vi "_Noise_YIG3.vi"(5 "Noise_YIG":T3={"Start(GHz)"=3.8, "Stop(GHz)"=12.2, "Step(GHz) "=0.2, "wait (S)"=0.1, "H/C SW"=0, "file_name"="", "P.M.aveg"=10, "save"=TRUE} {"H/C SW" items=["Liq Ni Motor", "NoiseSource Pow", "NoiseSource SP4T SW"]}, 6 "Bias_LO_equip":T1={"Node address"=19, "CAN Interface"="CAN1", "Cartridge band"=10, "Slave Node in"={"Address"=19, "Serial Number"=[16, 71, 55, 76, 1, 8, 0, -15]}, "ObjHandle out"=176554048, "POL"=1, "sb"=1, "GPIB_SM (SIS S,V)"="24", "GPIB_DMM (SIS I)"="22", "GPIB_SM (MAG I) "="25", "GPIB_SG(LO)"="19", "GPIB_PW (PAMP) "="6", "GPIB_TMP1(8ch)"="12", "GPIB_TMP2(2ch)  "="13", "WCA_avg"=10, "Rsen"=10.0, "BiasModule"=1, "LOModule "=5, "WCA_LO_FREQ_SET"={"YTO Low freq. [GHz]"=14.42, "YTO High freq. [GHz]"=17.7, "Kvco"=1, "Lock Pol."=0, "SET LO FREQ"=96.22222, "Multiplier"=6.0, "YTO (HEX)"=2014, "YTO ( FREQ)"=16.033167, "NULL PLL INTEGRATOR"=FALSE}, "Res for"=0} {"Res for" items=["none", "series res", "parallel res"]; "WCA_LO_FREQ_SET"."YTO ( FREQ)" min=25 max=150 step=0.0001 format="%.3f"; "WCA_LO_FREQ_SET"."Multiplier" min=3 max=6 step=3; "WCA_LO_FREQ_SET"."SET LO FREQ" min=25 max=150 step=0.0001 format="%.3f"; "WCA_LO_FREQ_SET"."Lock Pol." items=["Lower", "Upper"]; "WCA_LO_FREQ_SET"."Kvco" items=["7.5MHz/V", "15MHz/V"]; "WCA_LO_FREQ_SET"."YTO High freq. [GHz]" format="%.3f"; "WCA_LO_FREQ_SET"."YTO Low freq. [GHz]" format="%.3f"; "LOModule" items=["Manual Gunn+PAMP"=0, "PLL GUNN+PAMP"=5, "B10Lab LO"=1, "WCA LO"=2, ""=3, "YIG発信器"=4, "none"=99]; "BiasModule" items=["B10Lab Bias"=0, "WCA BiasModule"=1, "none"=99]; "Slave Node in"."Serial Number" format="%.0x"; "Slave Node in"."Address" format="%.0x"; "Cartridge band" max=10 step=1; "Node address" format="%.0x"}, 7 "Control":T2={"GPIB_ATT"="28", "6501Dev#"=1, "GPIB_SP"="18", "GPIB_PM"="13", "GPIB_DSA"="11", "GPIB_DMM (TPD)"="23", "GPIB_MPI"="2", "mortor設定"=[{"Axis"=0, "ID"=0, "HIspeed"=200.0, "LOspeed"=100.0, "ACCEL(ms)"=100.0, "Sratio"=50.0, "フリーラン\n"=FALSE, "文字列"="DSB HOT/COLD"}, {"Axis"=1, "ID"=0, "HIspeed"=4.0, "LOspeed"=4.0, "ACCEL(ms)"=100.0, "Sratio"=50.0, "フリーラン\n"=TRUE, "文字列"="SubMM Att"}, {"Axis"=0, "ID"=0, "HIspeed"=200.0, "LOspeed"=100.0, "ACCEL(ms)"=100.0, "Sratio"=50.0, "フリーラン\n"=TRUE, "文字列"="MPI Port1"}, {"Axis"=1, "ID"=0, "HIspeed"=200.0, "LOspeed"=100.0, "ACCEL(ms)"=100.0, "Sratio"=50.0, "フリーラン\n"=TRUE, "文字列"="MPI Port2"}], "DATAパス"=path "C:/Documents and Settings/?澤佳?/デスクトップ/data/プロトカ?トリッジ/100811_protC4-5/100904_P1_WCA_YIG", "DBパス "=path "Z:/band10/Labview_ALMA/MIX95/test", "comment"="100904_P1", "ColdCarts"="003601", "Th"=295.0, "Tc"=77.0, "Set_SIS_volt"=2.056451612903226, "Offset"=0.0, "control"=0, "FreqLO"=866.0, "Set_Mag_Cur"=800.0, "MPI offset(mm)"=22.986, "HOT/COLD"=0} {"HOT/COLD" items=["DSB", "SBR (Cart.)", "GainComp", "SBR (MIX)"]; "control" items=["CLOSE LOOP", "OPEN LOOP", "Not Control"]}) -> ()   [LabVIEW 2017]
uses:
  <vilib>/express/express arith-compare/Formula/XNode/ExpressFormulaBlockNode.xnode
panel:
  out "文字列":string
  in  "GPIB_NSPOW":string="4"
  out "XYグラフ 2":cluster{dbl[], dbl[]}(graph)={[3.8, 4.0, 4.2, 4.4, 4.6000000000000005, 4.800000000000001, 5.000000000000001, 5.200000000000001, 5.400000000000001, 5.600000000000001, 5.800000000000002, 6.000000000000002, 6.200000000000002, 6.400000000000002, 6.600000000000002, 6.8000000000000025, 7.000000000000003, 7.200000000000003, 7.400000000000003, 7.600000000000003, 7.800000000000003, 8.000000000000004, 8.200000000000003, 8.400000000000002, 8.600000000000001, 8.8, 9.0, 9.2, 9.399999999999999, 9.599999999999998, 9.799999999999997, 9.999999999999996, 10.199999999999996, 10.399999999999995, 10.599999999999994, 10.799999999999994, 10.999999999999993, 11.199999999999992, 11.399999999999991, 11.59999999999999, 11.79999999999999, 11.99999999999999, 12.199999999999989], [2162.2506307736817, 2610.001590658997, 3259.5497781050235, 2775.320412397087, 1731.9983281356488, 2481.779183137006, 2157.7510673198776, 1361.8845474426378, 682.5925239823699, 467.0395463865505, 435.3183157956642, 349.7678766673094, 257.35595108351663, 289.17415724926303, 272.2311885625452, 209.59141580739004, 206.53463871352125, 209.82364143887986, 193.6852217403505, 194.85552081739866, 186.2536165476463, 179.66627306574705, 180.29108492826452, 165.88232684665306, 170.21484313825314, 165.08707486423583, 161.69317508275617, 161.39594860807668, 157.61356167006898, 158.36459186549865, 162.3085451942526, 161.9946346155518, 165.27352115402942, 175.3117039214409, 165.6089313162741, 172.40460358258508, 178.15219547665433, 172.86473012765347, 183.70006104814289, 180.09761807812546, 191.78147420273163, 202.2277082874304, 182.5702492273905]}
  out "XYグラフ":cluster{dbl[], dbl[]}[](graph)=[{[3.8, 4.0, 4.2, 4.4, 4.6000000000000005, 4.800000000000001, 5.000000000000001, 5.200000000000001, 5.400000000000001, 5.600000000000001, 5.800000000000002, 6.000000000000002, 6.200000000000002, 6.400000000000002, 6.600000000000002, 6.8000000000000025, 7.000000000000003, 7.200000000000003, 7.400000000000003, 7.600000000000003, 7.800000000000003, 8.000000000000004, 8.200000000000003, 8.400000000000002, 8.600000000000001, 8.8, 9.0, 9.2, 9.399999999999999, 9.599999999999998, 9.799999999999997, 9.999999999999996, 10.199999999999996, 10.399999999999995, 10.599999999999994, 10.799999999999994, 10.999999999999993, 11.199999999999992, 11.399999999999991, 11.59999999999999, 11.79999999999999, 11.99999999999999, 12.199999999999989], [-12.6875455, -8.79275512, -6.28005577, -6.92868098, -8.7166628, -7.23493494, -7.37364738, -9.71131351, -11.7554011, -12.0808461, -12.5492271, -12.7463133, -13.372812, -14.3472225, -14.8493371, -15.5347475, -15.4508156, -15.5883011, -15.8732176, -15.6557263, -15.5366824, -16.038689, -16.8987194, -16.5991598, -17.7414209, -17.8823822, -17.4270802, -18.165907, -17.9285973, -17.7668847, -18.7346471, -18.8135922, -20.0978527, -20.2293386, -19.0504215, -19.9008061, -19.8130024, -19.1671194, -20.4106312, -20.1865464, -20.5863901, -22.2963949, -21.6268169]}, {[3.8, 4.0, 4.2, 4.4, 4.6000000000000005, 4.800000000000001, 5.000000000000001, 5.200000000000001, 5.400000000000001, 5.600000000000001, 5.800000000000002, 6.000000000000002, 6.200000000000002, 6.400000000000002, 6.600000000000002, 6.8000000000000025, 7.000000000000003, 7.200000000000003, 7.400000000000003, 7.600000000000003, 7.800000000000003, 8.000000000000004, 8.200000000000003, 8.400000000000002, 8.600000000000001, 8.8, 9.0, 9.2, 9.399999999999999, 9.599999999999998, 9.799999999999997, 9.999999999999996, 10.199999999999996, 10.399999999999995, 10.599999999999994, 10.799999999999994, 10.999999999999993, 11.199999999999992, 11.399999999999991, 11.59999999999999, 11.79999999999999, 11.99999999999999, 12.199999999999989], [-13.091013, -9.13153963, -6.55492569, -7.24853488, -9.21081505, -7.5900203, -7.77789058, -10.3239765, -12.851173, -13.5443165, -14.0889502, -14.53843, -15.5529118, -16.375769, -16.9558079, -17.9915143, -17.9277637, -18.0435485, -18.4388642, -18.2130248, -18.156679, -18.7088847, -19.5640687, -19.3811012, -20.4872111, -20.6710665, -20.2449254, -20.9863361, -20.7823418, -20.6139494, -21.5471582, -21.6288217, -22.8849531, -22.9338225, -21.8346772, -22.6286913, -22.4950179, -21.8912729, -23.0498547, -22.8533944, -23.1657372, -24.802363, -24.2746404]}]
  # "ENR21.8=>44183K"
  # "HOT/COLDのNoiseSourcePow\nはケンウッド電源のON/OFFのみ\n電圧は手動で設定する。"
  # "LO freq. [GHz]"
  # "YTO LOW\n/High Freq."
  # "ZERO Intgrtr"
  # "Node Address"
  # "Serial Number"
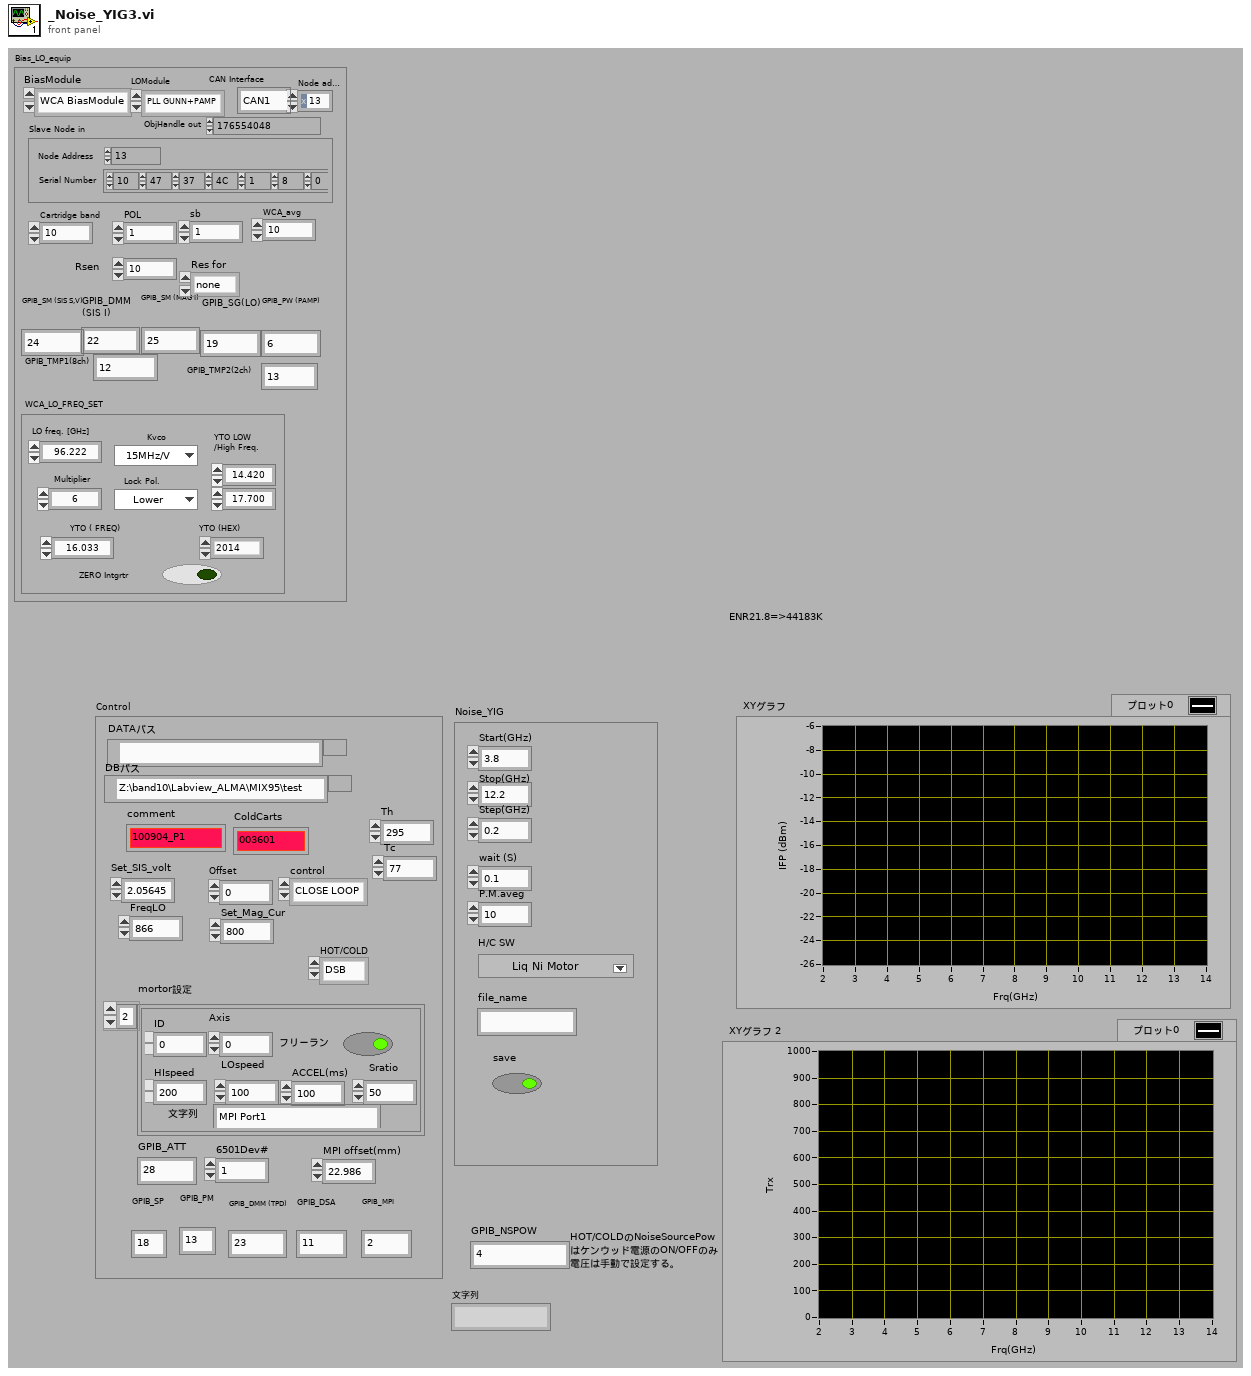
[diagram p1: front panel]
types:
  T1 = cluster{"Node address":u16, "CAN Interface":string, "Cartridge band":u32, "Slave Node in":cluster{"Address":i16, "Serial Number":i8[]}, "ObjHandle out":u32, "POL":u32, "sb":u32, "GPIB_SM (SIS S,V)":string, "GPIB_DMM (SIS I)":string, "GPIB_SM (MAG I) ":string, "GPIB_SG(LO)":string, "GPIB_PW (PAMP) ":string, "GPIB_TMP1(8ch)":string, "GPIB_TMP2(2ch)  ":string, "WCA_avg":i32, "Rsen":dbl, "BiasModule":u16, "LOModule ":u16, "WCA_LO_FREQ_SET":cluster{"YTO Low freq. [GHz]":sgl, "YTO High freq. [GHz]":sgl, "Kvco":u16, "Lock Pol.":u16, "SET LO FREQ":sgl, "Multiplier":sgl, "YTO (HEX)":u16, "YTO ( FREQ)":sgl, "NULL PLL INTEGRATOR":bool}, "Res for":u16}
  T2 = cluster{"GPIB_ATT":string, "6501Dev#":i16, "GPIB_SP":string, "GPIB_PM":string, "GPIB_DSA":string, "GPIB_DMM (TPD)":string, "GPIB_MPI":string, "mortor設定":cluster{"Axis":i16, "ID":i16, "HIspeed":dbl, "LOspeed":dbl, "ACCEL(ms)":dbl, "Sratio":dbl, "フリーラン\n":bool, "文字列":string}[], "DATAパス":path, "DBパス ":path, "comment":string, "ColdCarts":string, "Th":dbl, "Tc":dbl, "Set_SIS_volt":dbl, "Offset":dbl, "control":u16, "FreqLO":dbl, "Set_Mag_Cur":dbl, "MPI offset(mm)":dbl, "HOT/COLD":u16}
  T3 = cluster{"Start(GHz)":dbl, "Stop(GHz)":dbl, "Step(GHz) ":dbl, "wait (S)":dbl, "H/C SW":u16, "file_name":string, "P.M.aveg":i32, "save":bool}
  T4 = cluster{"Axis":i16, "ID":i16, "HIspeed":dbl, "LOspeed":dbl, "ACCEL(ms)":dbl, "Sratio":dbl, "フリーラン\n":bool, "文字列":string}[]
  T5 = cluster{"Axis":i16, "ID":i16, "HIspeed":dbl, "LOspeed":dbl, "ACCEL(ms)":dbl, "Sratio":dbl, "フリーラン\n":bool, "文字列":string}
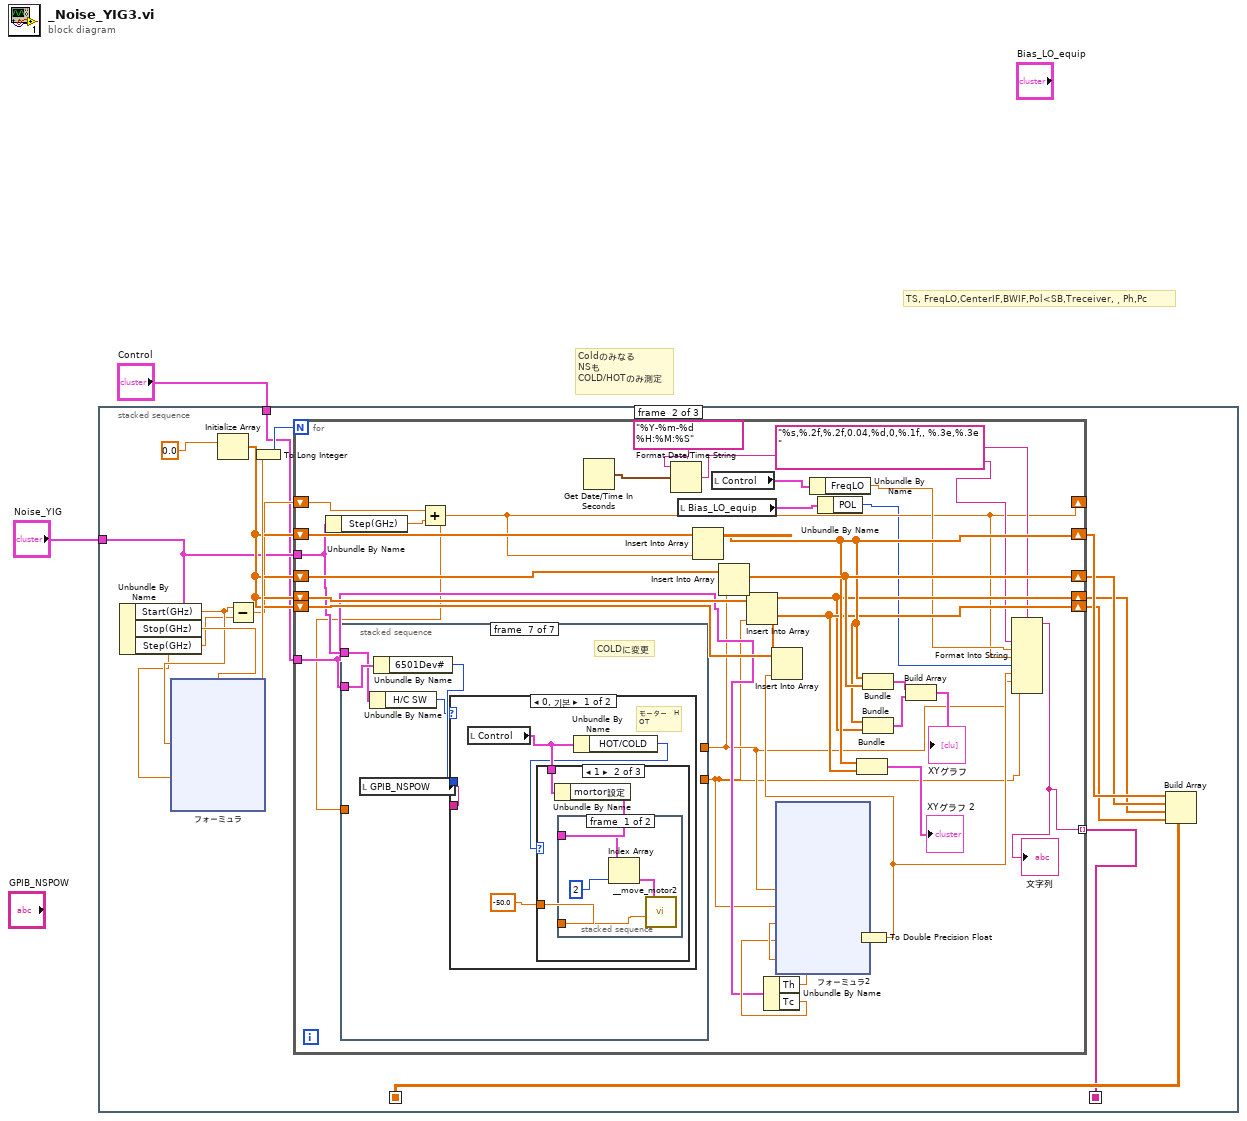
[diagram p0: block diagram]
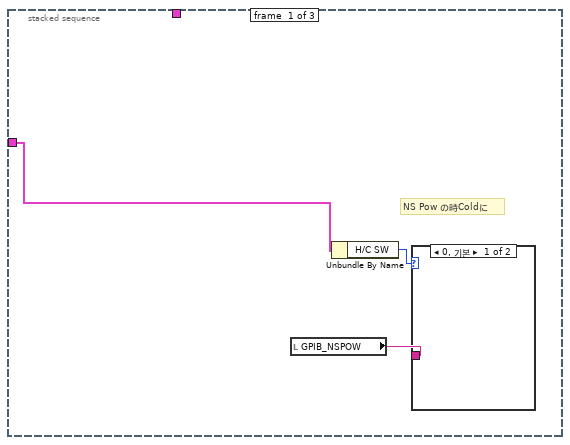
[diagram p2: hidden frame]
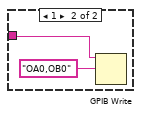
[diagram p3: hidden frame]
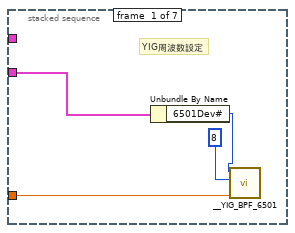
[diagram p4: hidden frame]
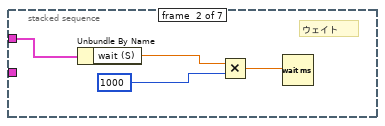
[diagram p5: hidden frame]
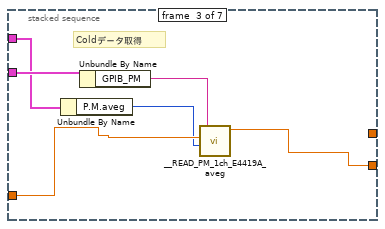
[diagram p6: hidden frame]
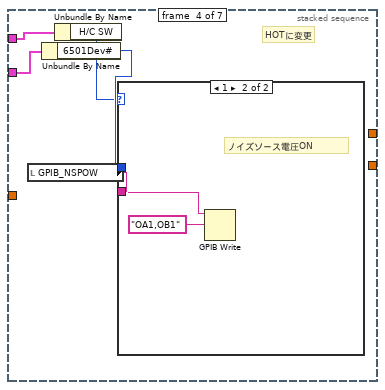
[diagram p7: hidden frame]
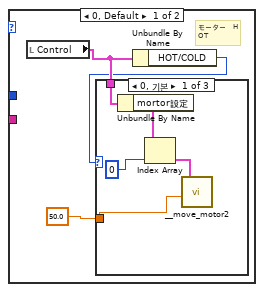
[diagram p8: hidden frame]
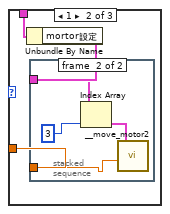
[diagram p9: hidden frame]
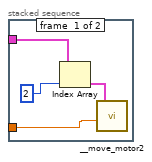
[diagram p10: hidden frame]
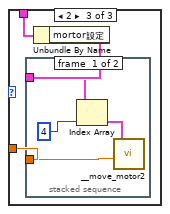
[diagram p11: hidden frame]
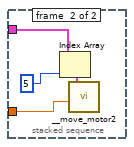
[diagram p12: hidden frame]
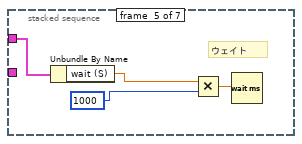
[diagram p13: hidden frame]
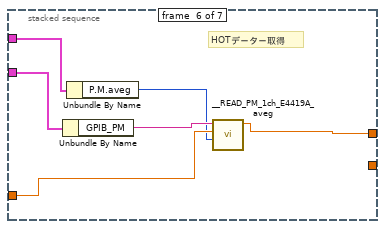
[diagram p14: hidden frame]
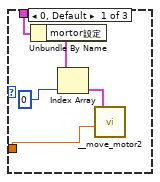
[diagram p15: hidden frame]
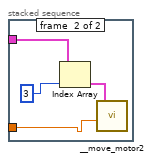
[diagram p16: hidden frame]
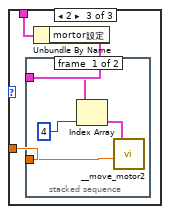
[diagram p17: hidden frame]
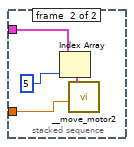
[diagram p18: hidden frame]
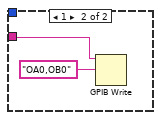
[diagram p19: hidden frame]
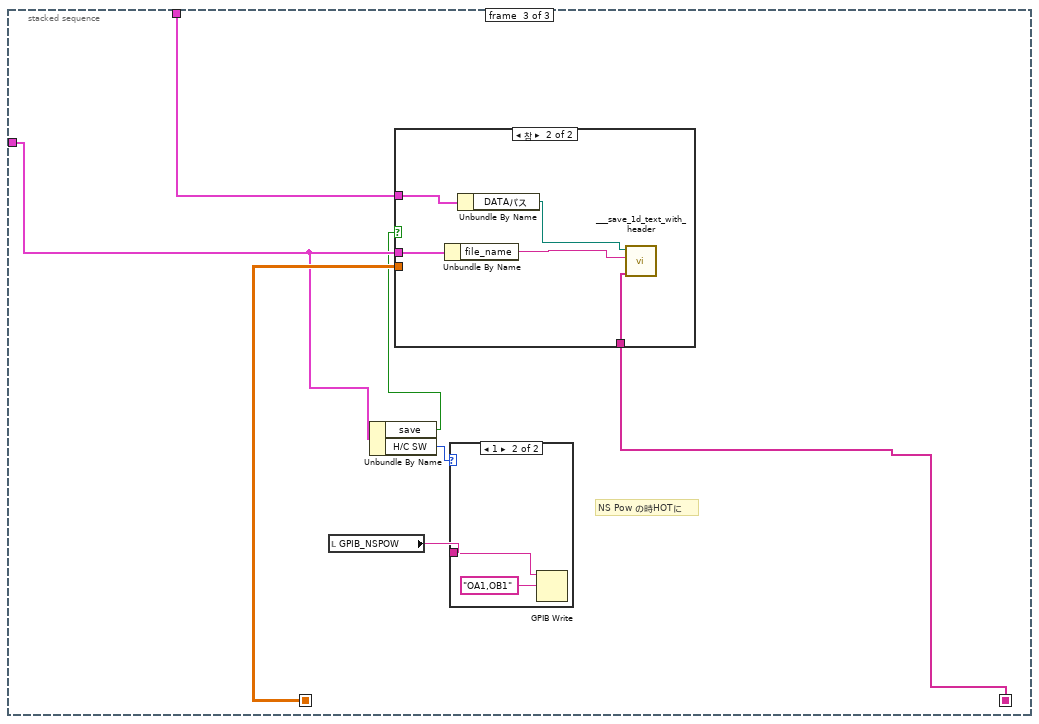
[diagram p20: hidden frame]
diagram:
  # "TS, FreqLO,CenterIF,BWIF,Pol<SB,Treceiver,，Ph,Pc"
  # "Coldのみなる\nNSも\nCOLD/HOTのみ測定"
  n1 = stacked-sequence {
    seq-local: [_ w10 _] -> [_ _ w186]
    seq-local: [_ w8 _] -> [_ _ w180]
    tunnel: "Noise_YIG" -> [w3 w15 w182]
    tunnel: "Control" -> [_ w9 w185]
    frame #0 {
      # "NS Pow の時Coldに"
      n2 = local read "GPIB_NSPOW"() -> (w5:string)
      n3 = Unbundle By Name(w3) -> ("H/C SW"=w4:u16)
      n4 = case shown="0, 기본" w4 {
        tunnel: w5 -> [_ w6]
        frame 0, Default {
        }
        frame 1 {
          n5 = GPIB Write(0:w6, 1:"OA0,OB0") -> ()  [unwired: 3 in, 2 out]
        }
      }
    }
    frame #1 {
      n6 = Unbundle By Name(w15) -> ("Start(GHz)"=w18:dbl, "Stop(GHz)"=w22:dbl, "Step(GHz)"=w17:dbl)
      n7 = xnode "フォーミュラ"("start"=w18, "stop"=w22, "step"=w17) -> ("結果"=w23:dbl)  [unwired: 1 in, 1 out]
      n8 = Initialize Array(0.0) -> (w20:dbl[])  [unwired: 1 in]
      n9 = Subtract(x=w18, y=w17) -> (x-y=w19:dbl)
      n10 = To Long Integer(number=w23) -> (32bit integer=w16:i32)
      n11 = for {
        N: w16 -> [_]
        shift-right: [w41] -> _
        shift-left: w19 -> [w54]
        tunnel: w15 -> [w50]
        shift-right: [w59] -> w13
        shift-left: w20 -> [w66]
        shift-right: [w58] -> w14
        shift-left: w20 -> [w65]
        shift-right: [w53] -> w12
        shift-left: w20 -> [w64]
        shift-right: [w57] -> w11
        shift-left: w20 -> [w63]
        tunnel: w9 -> [w49]
        tunnel: [w40] -> w8 mode=indexing
        n12 = Unbundle By Name(w50) -> ("Step(GHz)"=w67:dbl)
        n13 = Add(x=w54, y=w67) -> (x+y=w41:dbl)
        n14 = stacked-sequence {
          tunnel: w49 -> [w82 _ w95 w100 _ w142 w147]
          tunnel: [_ _ _ _ _ w137 _] -> w37
          tunnel: [_ _ w90 _ _ _ _] -> w36
          tunnel: w41 -> [w83 _ w93 _ _ w140 _]
          tunnel: w50 -> [_ w86 w92 w97 w133 w139 w144]
          frame #0 {
            # "YIG周波数設定"
            n15 = Unbundle By Name(w82) -> ("6501Dev#"=w84:i16)
            n16 = call "__YIG_BPF_6501.vi"("fc(GHz)"=w83, "bit"=8, "Dev(1,2..)"=w84) -> ()  [unwired: 1 in]
          }
          frame #1 {
            # "ウェイト"
            n17 = Unbundle By Name(w86) -> ("wait (S)"=w89:dbl)
            n18 = Multiply(x=w89, y=1000) -> (x*y=w87:dbl)
            n19 = Wait (ms)(milliseconds to wait=w87) -> ()  [unwired: 1 out]
          }
          frame #2 {
            # "Coldデータ取得"
            n20 = Unbundle By Name(w92) -> ("P.M.aveg"=w91:i32)
            n21 = Unbundle By Name(w95) -> ("GPIB_PM"=w94:string)
            n22 = call "__READ_PM_1ch_E4419A_aveg.VI"("aveg"=w91, "frq(GHz)"=w93, "GPIB"=w94) -> ("chA"=w90:dbl)  [unwired: 4 in]
          }
          frame #3 {
            # "HOTに変更"
            n23 = local read "GPIB_NSPOW"() -> (w98:string)
            n24 = Unbundle By Name(w100) -> ("6501Dev#"=w99:i16)
            n25 = Unbundle By Name(w97) -> ("H/C SW"=w96:u16)
            n26 = case shown="1" w96 {
              tunnel: w99 -> [_ _]
              tunnel: w98 -> [_ w131]
              frame 0, Default {
                # "モーター　HOT"
                n27 = local read "Control"() -> (w103:T2)
                n28 = Unbundle By Name(w103) -> ("HOT/COLD"=w102:u16)
                n29 = case shown="0, 기본" w102 {
                  tunnel: w103 -> [w107 w111 w122]
                  tunnel: 50.0 -> [w104 w109 w120]
                  frame 0, Default {
                    n30 = Unbundle By Name(w107) -> ("mortor設定"=w106:T4)
                    n31 = Index Array(array=w106, index=0) -> (element=w105:T5)
                    n32 = call "__move_motor2.vi"("Moving distance"=w104, "motor setup"=w105) -> ()  [unwired: 2 in, 2 out]
                  }
                  frame 1 {
                    n33 = Unbundle By Name(w111) -> ("mortor設定"=w110:T4)
                    n34 = stacked-sequence {
                      tunnel: w110 -> [w114 w118]
                      tunnel: w109 -> [w112 w116]
                      frame #0 {
                        n35 = Index Array(array=w114, index=2) -> (element=w113:T5)
                        n36 = call "__move_motor2.vi"("Moving distance"=w112, "motor setup"=w113) -> ()  [unwired: 2 in, 2 out]
                      }
                      frame #1 {
                        n37 = Index Array(array=w118, index=3) -> (element=w117:T5)
                        n38 = call "__move_motor2.vi"("Moving distance"=w116, "motor setup"=w117) -> ()  [unwired: 2 in, 2 out]
                      }
                    }
                  }
                  frame 2 {
                    n39 = Unbundle By Name(w122) -> ("mortor設定"=w121:T4)
                    n40 = stacked-sequence {
                      tunnel: w121 -> [w125 w129]
                      tunnel: w120 -> [w123 w127]
                      frame #0 {
                        n41 = Index Array(array=w125, index=4) -> (element=w124:T5)
                        n42 = call "__move_motor2.vi"("Moving distance"=w123, "motor setup"=w124) -> ()  [unwired: 2 in, 2 out]
                      }
                      frame #1 {
                        n43 = Index Array(array=w129, index=5) -> (element=w128:T5)
                        n44 = call "__move_motor2.vi"("Moving distance"=w127, "motor setup"=w128) -> ()  [unwired: 2 in, 2 out]
                      }
                    }
                  }
                }
              }
              frame 1 {
                # "ノイズソース電圧ON"
                n45 = GPIB Write(0:w131, 1:"OA1,OB1") -> ()  [unwired: 3 in, 2 out]
              }
            }
          }
          frame #4 {
            # "ウェイト"
            n46 = Unbundle By Name(w133) -> ("wait (S)"=w136:dbl)
            n47 = Multiply(x=w136, y=1000) -> (x*y=w134:dbl)
            n48 = Wait (ms)(milliseconds to wait=w134) -> ()  [unwired: 1 out]
          }
          frame #5 {
            # "HOTデーター取得"
            n49 = Unbundle By Name(w142) -> ("GPIB_PM"=w141:string)
            n50 = Unbundle By Name(w139) -> ("P.M.aveg"=w138:i32)
            n51 = call "__READ_PM_1ch_E4419A_aveg.VI"("aveg"=w138, "frq(GHz)"=w140, "GPIB"=w141) -> ("chA"=w137:dbl)  [unwired: 4 in]
          }
          frame #6 {
            # "COLDに変更"
            n52 = local read "GPIB_NSPOW"() -> (w145:string)
            n53 = Unbundle By Name(w144) -> ("H/C SW"=w143:u16)
            n54 = Unbundle By Name(w147) -> ("6501Dev#"=w146:i16)
            n55 = case shown="0, 기본" w143 {
              tunnel: w146 -> [_ _]
              tunnel: w145 -> [_ w178]
              frame 0, Default {
                # "モーター　HOT"
                n56 = local read "Control"() -> (w150:T2)
                n57 = Unbundle By Name(w150) -> ("HOT/COLD"=w149:u16)
                n58 = case shown="1" w149 {
                  tunnel: w150 -> [w154 w158 w169]
                  tunnel: -50.0 -> [w151 w156 w167]
                  frame 0, Default {
                    n59 = Unbundle By Name(w154) -> ("mortor設定"=w153:T4)
                    n60 = Index Array(array=w153, index=0) -> (element=w152:T5)
                    n61 = call "__move_motor2.vi"("Moving distance"=w151, "motor setup"=w152) -> ()  [unwired: 2 in, 2 out]
                  }
                  frame 1 {
                    n62 = Unbundle By Name(w158) -> ("mortor設定"=w157:T4)
                    n63 = stacked-sequence {
                      tunnel: w157 -> [w161 w165]
                      tunnel: w156 -> [w159 w163]
                      frame #0 {
                        n64 = Index Array(array=w161, index=2) -> (element=w160:T5)
                        n65 = call "__move_motor2.vi"("Moving distance"=w159, "motor setup"=w160) -> ()  [unwired: 2 in, 2 out]
                      }
                      frame #1 {
                        n66 = Index Array(array=w165, index=3) -> (element=w164:T5)
                        n67 = call "__move_motor2.vi"("Moving distance"=w163, "motor setup"=w164) -> ()  [unwired: 2 in, 2 out]
                      }
                    }
                  }
                  frame 2 {
                    n68 = Unbundle By Name(w169) -> ("mortor設定"=w168:T4)
                    n69 = stacked-sequence {
                      tunnel: w168 -> [w172 w176]
                      tunnel: w167 -> [w170 w174]
                      frame #0 {
                        n70 = Index Array(array=w172, index=4) -> (element=w171:T5)
                        n71 = call "__move_motor2.vi"("Moving distance"=w170, "motor setup"=w171) -> ()  [unwired: 2 in, 2 out]
                      }
                      frame #1 {
                        n72 = Index Array(array=w176, index=5) -> (element=w175:T5)
                        n73 = call "__move_motor2.vi"("Moving distance"=w174, "motor setup"=w175) -> ()  [unwired: 2 in, 2 out]
                      }
                    }
                  }
                }
              }
              frame 1 {
                n74 = GPIB Write(0:w178, 1:"OA0,OB0") -> ()  [unwired: 3 in, 2 out]
              }
            }
          }
        }
        n75 = Get Date/Time In Seconds() -> (seconds since 1Jan1904=w48:timestamp)
        n76 = Format Date/Time String(time format string (%c)="%Y-%m-%d  %H:%M:%S", seconds (now)=w48) -> (date/time string=w43:string)  [unwired: 1 in]
        n77 = local read "Bias_LO_equip"() -> (w45:T1)
        n78 = Insert Into Array(array=w65, new element=w41) -> (w58:dbl[])  [unwired: 1 in]
        n79 = local read "Control"() -> (w46:T2)
        n80 = Insert Into Array(array=w66, new element=w37) -> (w59:dbl[])  [unwired: 1 in]
        n81 = Insert Into Array(array=w64, new element=w36) -> (w53:dbl[])  [unwired: 1 in]
        n82 = Unbundle By Name(w49) -> ("Th"=w52:dbl, "Tc"=w51:dbl)
        n83 = xnode "フォーミュラ2"("ph"=w37, "pc"=w36, "th"=w52, "tc"=w51) -> ("結果"=w62:dbl)  [unwired: 1 in, 1 out]
        n84 = Unbundle By Name(w46) -> ("FreqLO"=w42:dbl)
        n85 = Unbundle By Name(w45) -> ("POL"=w39:u32)
        n86 = To Double Precision Float(number=w62) -> (double precision float=w38:dbl)
        n87 = Insert Into Array(array=w63, new element=w38) -> (w57:dbl[])  [unwired: 1 in]
        n88 = Bundle "Bundle"(w58, w57) -> (→"XYグラフ 2":cluster{dbl[], dbl[]})  [unwired: 1 in]
        n89 = Bundle "Bundle"(w58, w59) -> (w60:cluster{dbl[], dbl[]})  [unwired: 1 in]
        n90 = Bundle "Bundle"(w58, w53) -> (w61:cluster{dbl[], dbl[]})  [unwired: 1 in]
        n91 = Build Array "Build Array"(w60, w61) -> (→"XYグラフ":cluster{dbl[], dbl[]}[])
        n92 = Format Into String(format string="%s,%.2f,%.2f,0.04,%d,0,%.1f,, %.3e,%.3e ", w43, w42, w41, w39, w38, w37, w36) -> (resulting string=w40:string)  [unwired: 2 in, 1 out]
        "文字列" <- w40
      }
      n93 = Build Array(w14, w13, w12, w11) -> (w10:dbl[][])
    }
    frame #2 {
      # "NS Pow の時HOTに"
      n94 = local read "GPIB_NSPOW"() -> (w184:string)
      n95 = Unbundle By Name(w182) -> ("save"=w181:bool, "H/C SW"=w183:u16)
      n96 = case shown="참" w181 {
        tunnel: w186 -> [_ _]
        tunnel: w185 -> [_ w191]
        tunnel: w182 -> [_ w190]
        tunnel: w180 -> [_ w187]
        frame False {
        }
        frame True {
          n97 = Unbundle By Name(w190) -> ("file_name"=w188:string)
          n98 = Unbundle By Name(w191) -> ("DATAパス"=w189:path)
          n99 = call "___save_1d_text_with_header.vi"("配列"=w187, "file_name"=w188, "パス"=w189) -> ()  [unwired: 8 in, 1 out]
        }
      }
      n100 = case shown="1" w183 {
        tunnel: w184 -> [_ w192]
        frame 0, Default {
        }
        frame 1 {
          n101 = GPIB Write(0:w192, 1:"OA1,OB1") -> ()  [unwired: 3 in, 2 out]
        }
      }
    }
  }
